vi "Get Jacobian.vi"(8 "error in (no error)":errorcluster, 11 "Finger in":refnum<class "Finger.lvclass">) -> (0 "error out":errorcluster, 2 "Jacobian":T1, 3 "Finger out":refnum<class "Finger.lvclass">)   [LabVIEW 2013, in "Finger.lvclass"]
uses:
  Finger.lvclass
  <vilib>/Analysis/Matrix/Datatypes/RealMatrix.ctl
  Finger.lvclass/Finger.ctl
  <vilib>/Analysis/Matrix/Numeric/Multiply/Multiply - RM,RM.vi
  <vilib>/Analysis/Matrix/Numeric/Conversions/Array To Matrix - RA.vi
  <vilib>/Analysis/Matrix/NI_Matrix.lvlib
  <vilib>/robotics/Kinematics/NI_Kinematics.lvlib
  <vilib>/Analysis/NI_AALPro.lvlib
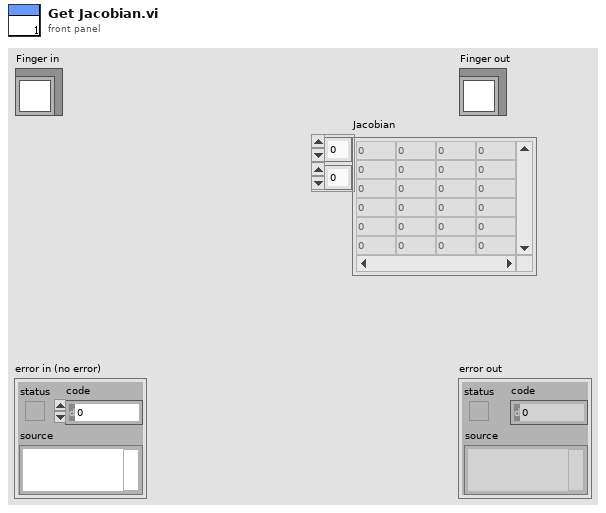
[diagram p1: front panel]
types:
  T1 = typedef "NI_Matrix.lvlib/RealMatrix.ctl" = dbl[][]
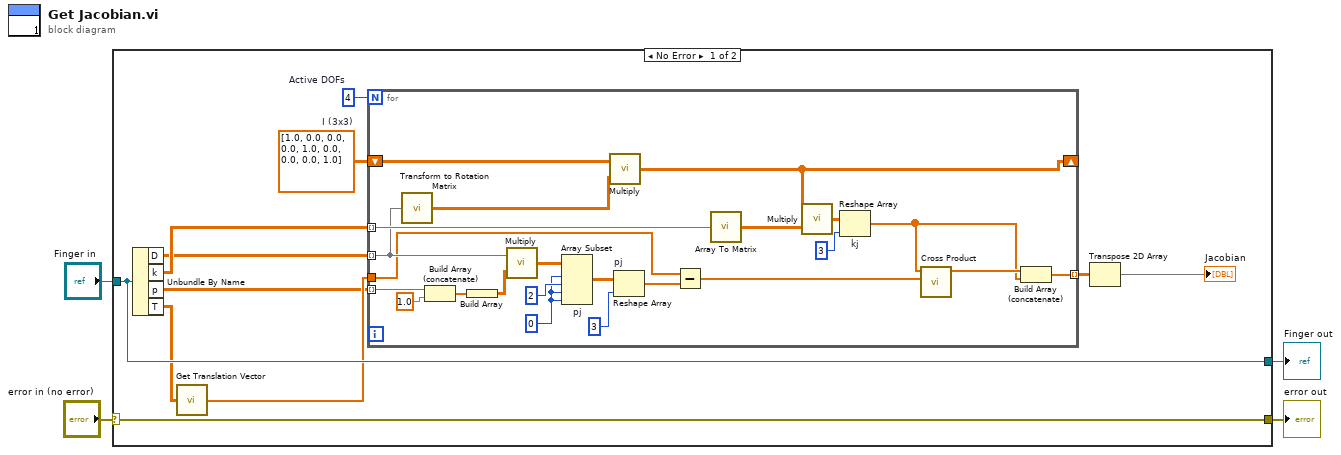
[diagram p0: block diagram]
diagram:
  n1 = case shown="No Error" "error in (no error)" {
    selector: "error in (no error)" -> [w15 w40]
    tunnel: [w15 w40] -> w3
    tunnel: [w14 w39] -> w1
    tunnel: "Finger in" -> [w14 w39]
    frame No Error {
      w5 = T1 [[1.0, 0.0, 0.0], [0.0, 1.0, 0.0], [0.0, 0.0, 1.0]]  # I (3x3)
      w13 = 4  # Active DOFs
      n2 = Unbundle By Name(w14) -> ("D"=w7:dbl[][][], "k"=w8:T1, "p"=w9:T1, "T"=w6:T1)
      n3 = call <vilib>:"Get Translation Vector.vi"("transform"=w6) -> ("translation vector"=w12:dbl[])
      n4 = for {
        N: w13 -> [_]
        tunnel: w7 -> [w33] mode=indexing
        shift-right: [w36] -> _
        shift-left: w5 -> [w38]
        tunnel: w8 -> [w34] mode=indexing
        tunnel: w9 -> [w18] mode=indexing
        tunnel: w12 -> [w29]
        tunnel: [w20] -> w11 mode=indexing
        w30 = 0 ("row 1")
        n5 = call <vilib>:"Transform to Rotation Matrix.vi"("transform"=w33) -> ("rotation matrix"=w37:T1)
        n6 = Build Array (concatenate)(w18, 1.0) -> (w17:dbl[])
        n7 = Build Array(w17) -> (w19:T1)
        n8 = call-poly <vilib>:"Multiply.vi"("Real Matrix B"=w19, "Real Matrix A"=w33) -> ("A * B"=w32:T1)
        n9 = Array Subset "pj"(array=w32, index (row)=w30, length (row)=2 ("row N"), index (col)=w30, length (col)=w30) -> (w28:T1)
        n10 = call-poly <vilib>:"Multiply.vi"("Real Matrix B"=w37, "Real Matrix A"=w38) -> ("A * B"=w36:T1)
        n11 = Reshape Array "pj"(w28, 3 ("dimension size")) -> (w26:dbl[])
        n12 = Subtract(x=w29, y=w26) -> (x-y=w23:dbl[])
        n13 = call-poly <vilib>:"Array To Matrix.vi"("Real 1D Array"=w34) -> ("Real Matrix (Column Vector)"=w35:T1)
        n14 = call-poly <vilib>:"Multiply.vi"("Real Matrix B"=w35, "Real Matrix A"=w36) -> ("A * B"=w24:T1)
        n15 = Reshape Array "kj"(w24, 3 ("dimension size")) -> (w21:dbl[])
        n16 = call <vilib>:"Cross Product.vi"("B Vector"=w23, "A Vector"=w21) -> ("Cross Product"=w22:dbl[])  [unwired: 8 in, 1 out]
        n17 = Build Array (concatenate)(w22, w21) -> (w20:dbl[])
      }
      n18 = Transpose 2D Array(2D array=w11) -> (transposed array=→"Jacobian":dbl[][])
    }
    frame Error {
    }
  }
  "error out" <- w3
  "Finger out" <- w1
